vi "test-rotation2d.vi"(8 "error in (no error)":errorcluster) -> (0 "error out":errorcluster, 3 "ALL TESTS PASSED":bool)   [LabVIEW 2019]
uses:
  <vilib>/Rock Robotics/WPI/ThirdParty/JAS_Junk/TrajLib/Rotation2d_Plus.vi
  <vilib>/Rock Robotics/WPI/ThirdParty/JAS_Junk/TrajLib/MathUtil_Clamp.vi
  <vilib>/Rock Robotics/WPI/ThirdParty/JAS_Junk/TrajLib/Rotation2d_Times.vi
  <vilib>/Rock Robotics/WPI/ThirdParty/JAS_Junk/TrajLib/Util_CalcDist.vi
  <vilib>/Rock Robotics/WPI/ThirdParty/JAS_Junk/TrajLib/Rotation2d_UnaryMinus.vi
  <vilib>/Rock Robotics/WPI/ThirdParty/JAS_Junk/TrajLib/Rotation2d_CreateXY.vi
  <vilib>/Rock Robotics/WPI/ThirdParty/JAS_Junk/TrajLib/Trajectory_Library.lvlib
panel:
  out "T9 - True":bool
  out "T8 - True":bool
  out "T7 - True":bool
  out "T4 -- X -- 0":dbl
  out "T3 -- X -- 0":dbl
  out "T2 -- y -- 0":dbl
  out "T2 -- X -- 0":dbl
  out "T6 - False":bool
  out "T5 - True":bool
  out "T1 -- y -- 0":dbl
  out "T1 -- X -- 0":dbl
  out "T0 -- y -- 0":dbl
  out "T0 -- X -- 0":dbl
  # "Rotation2D Test"
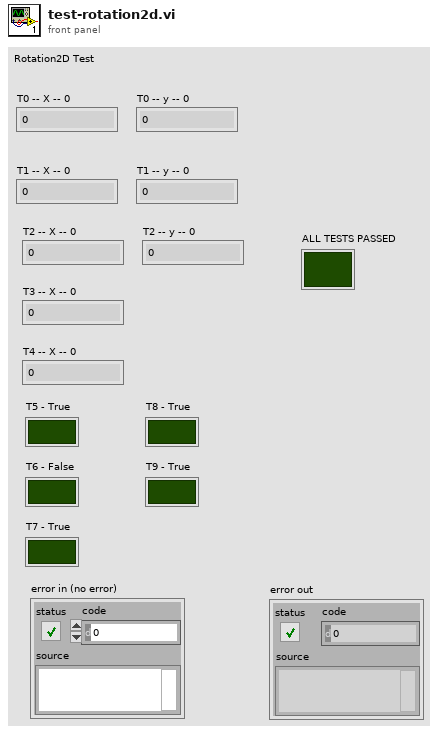
[diagram p1: front panel]
types:
  T1 = typedef "Trajectory_Library.lvlib/ROTATION2D.ctl" = cluster{"VALUE":dbl, "COS":dbl, "SIN":dbl}
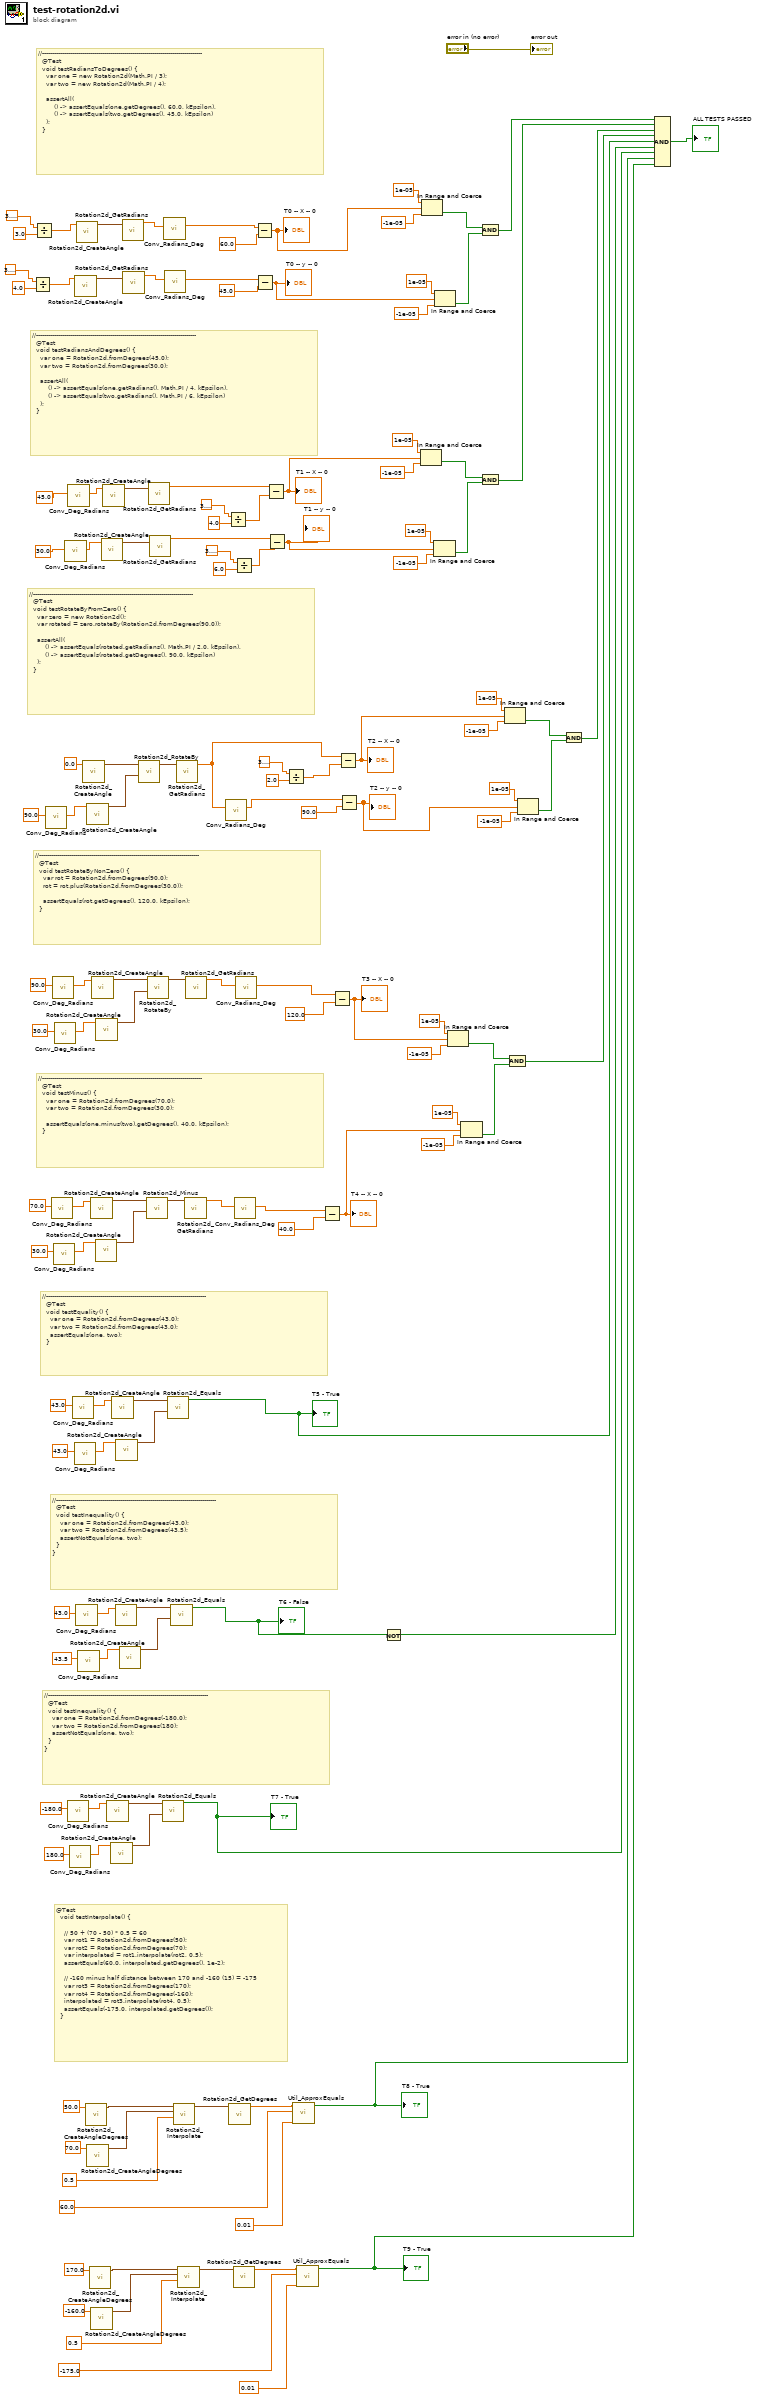
[diagram p0: block diagram]
diagram:
  # "@Test\n  void testInterpolate() {\n\n    // 50 + (70 - 50) * 0.5 = 60\n    var rot1 = Rotation2d.fromDegrees(50);\n    var rot2 = Rotation2d.fromDegrees(70);\n    var interpolated = rot1.interpolate(rot2, 0.5);\n    assertEquals(60.0, interpolated.getDegrees(), 1e-2);\n\n    // -160 minus half distance between 170 and -160 (15) = -175\n    var rot3 = Rotation2d.fromDegrees(170);\n    var rot4 = Rotation2d.fromDegrees(-160);\n    interpolated = rot3.interpolate(rot4, 0.5);\n    assertEquals(-175.0, interpolated.getDegrees());\n  }"
  # "//--------------------------------------------------------------------------------\n  @Test\n  void testInequality() {\n    var one = Rotation2d.fromDegrees(-180.0);\n    var two = Rotation2d.fromDegrees(180);\n    assertNotEquals(one, two);\n  }\n}"
  # "//--------------------------------------------------------------------------------\n  @Test\n  void testInequality() {\n    var one = Rotation2d.fromDegrees(43.0);\n    var two = Rotation2d.fromDegrees(43.5);\n    assertNotEquals(one, two);\n  }\n}"
  # "//--------------------------------------------------------------------------------\n  @Test\n  void testMinus() {\n    var one = Rotation2d.fromDegrees(70.0);\n    var two = Rotation2d.fromDegrees(30.0);\n\n    assertEquals(one.minus(two).getDegrees(), 40.0, kEpsilon);\n  }"
  # "//--------------------------------------------------------------------------------\n  @Test\n  void testRotateByNonZero() {\n    var rot = Rotation2d.fromDegrees(90.0);\n    rot = rot.plus(Rotation2d.fromDegrees(30.0));\n\n    assertEquals(rot.getDegrees(), 120.0, kEpsilon);\n  }"
  # "//--------------------------------------------------------------------------------\n  @Test\n  void testRotateByFromZero() {\n    var zero = new Rotation2d();\n    var rotated = zero.rotateBy(Rotation2d.fromDegrees(90.0));\n\n    assertAll(\n        () -> assertEquals(rotated.getRadians(), Math.PI / 2.0, kEpsilon),\n        () -> assertEquals(rotated.getDegrees(), 90.0, kEpsilon)\n    );\n  }"
  # "//--------------------------------------------------------------------------------\n  @Test\n  void testEquality() {\n    var one = Rotation2d.fromDegrees(43.0);\n    var two = Rotation2d.fromDegrees(43.0);\n    assertEquals(one, two);\n  }"
  # "//--------------------------------------------------------------------------------\n  @Test\n  void testRadiansAndDegrees() {\n    var one = Rotation2d.fromDegrees(45.0);\n    var two = Rotation2d.fromDegrees(30.0);\n\n    assertAll(\n        () -> assertEquals(one.getRadians(), Math.PI / 4, kEpsilon),\n        () -> assertEquals(two.getRadians(), Math.PI / 6, kEpsilon)\n    );\n  }"
  # "//--------------------------------------------------------------------------------\n  @Test\n  void testRadiansToDegrees() {\n    var one = new Rotation2d(Math.PI / 3);\n    var two = new Rotation2d(Math.PI / 4);\n\n    assertAll(\n        () -> assertEquals(one.getDegrees(), 60.0, kEpsilon),\n        () -> assertEquals(two.getDegrees(), 45.0, kEpsilon)\n    );\n  }"
  n1 = Divide(x=3.141592653589793, y=4.0) -> (x/y=w128:dbl)
  n2 = Divide(x=3.141592653589793, y=3.0) -> (x/y=w131:dbl)
  n3 = call <vilib>:"Conv_Deg_Radians.vi"("Degress"=90.0) -> ("Radians"=w137:dbl)  [unwired: 10 in]
  n4 = call <vilib>:"Conv_Deg_Radians.vi"("Degress"=70.0) -> ("Radians"=w82:dbl)  [unwired: 10 in]
  n5 = call <vilib>:"Conv_Deg_Radians.vi"("Degress"=90.0) -> ("Radians"=w91:dbl)  [unwired: 10 in]
  n6 = call <vilib>:"Conv_Deg_Radians.vi"("Degress"=30.0) -> ("Radians"=w89:dbl)  [unwired: 10 in]
  n7 = call <vilib>:"Conv_Deg_Radians.vi"("Degress"=30.0) -> ("Radians"=w98:dbl)  [unwired: 10 in]
  n8 = call <vilib>:"Conv_Deg_Radians.vi"("Degress"=30.0 ("y")) -> ("Radians"=w113:dbl)  [unwired: 10 in]
  n9 = call <vilib>:"Conv_Deg_Radians.vi"("Degress"=-180.0) -> ("Radians"=w63:dbl)  [unwired: 10 in]
  n10 = call <vilib>:"Conv_Deg_Radians.vi"("Degress"=45.0 ("y")) -> ("Radians"=w112:dbl)  [unwired: 10 in]
  n11 = call <vilib>:"Conv_Deg_Radians.vi"("Degress"=180.0) -> ("Radians"=w68:dbl)  [unwired: 10 in]
  n12 = call <vilib>:"Conv_Deg_Radians.vi"("Degress"=43.0) -> ("Radians"=w75:dbl)  [unwired: 10 in]
  n13 = call <vilib>:"Conv_Deg_Radians.vi"("Degress"=43.0) -> ("Radians"=w80:dbl)  [unwired: 10 in]
  n14 = call <vilib>:"Rotation2d_CreateAngle.vi"("Angle"=w128) -> ("ROTATION"=w124:T1)  [unwired: 10 in]
  n15 = call <vilib>:"Conv_Deg_Radians.vi"("Degress"=43.0) -> ("Radians"=w69:dbl)  [unwired: 10 in]
  n16 = call <vilib>:"Rotation2d_CreateAngle.vi"("Angle"=w131) -> ("ROTATION"=w127:T1)  [unwired: 10 in]
  n17 = call <vilib>:"Conv_Deg_Radians.vi"("Degress"=43.5) -> ("Radians"=w74:dbl)  [unwired: 10 in]
  n18 = call <vilib>:"Rotation2d_CreateAngle.vi"("Angle"=0.0) -> ("ROTATION"=w106:T1)  [unwired: 10 in]
  n19 = call <vilib>:"Rotation2d_CreateAngleDegrees.vi"("Angle_Degrees"=50.0) -> ("ROTATION"=w18:T1)  [unwired: 10 in]
  n20 = call <vilib>:"Rotation2d_CreateAngle.vi"("Angle"=w137) -> ("ROTATION"=w105:T1)  [unwired: 10 in]
  n21 = call <vilib>:"Rotation2d_CreateAngleDegrees.vi"("Angle_Degrees"=70.0) -> ("ROTATION"=w17:T1)  [unwired: 10 in]
  n22 = call <vilib>:"Rotation2d_CreateAngleDegrees.vi"("Angle_Degrees"=170.0) -> ("ROTATION"=w9:T1)  [unwired: 10 in]
  n23 = call <vilib>:"Rotation2d_CreateAngle.vi"("Angle"=w82) -> ("ROTATION"=w87:T1)  [unwired: 10 in]
  n24 = call <vilib>:"Rotation2d_CreateAngleDegrees.vi"("Angle_Degrees"=-160.0) -> ("ROTATION"=w8:T1)  [unwired: 10 in]
  n25 = call <vilib>:"Rotation2d_CreateAngle.vi"("Angle"=w91) -> ("ROTATION"=w96:T1)  [unwired: 10 in]
  n26 = call <vilib>:"Rotation2d_CreateAngle.vi"("Angle"=w89) -> ("ROTATION"=w86:T1)  [unwired: 10 in]
  n27 = call <vilib>:"Rotation2d_CreateAngle.vi"("Angle"=w98) -> ("ROTATION"=w95:T1)  [unwired: 10 in]
  n28 = call <vilib>:"Rotation2d_CreateAngle.vi"("Angle"=w113) -> ("ROTATION"=w120:T1)  [unwired: 10 in]
  n29 = call <vilib>:"Rotation2d_CreateAngle.vi"("Angle"=w112) -> ("ROTATION"=w121:T1)  [unwired: 10 in]
  n30 = call <vilib>:"Rotation2d_CreateAngle.vi"("Angle"=w63) -> ("ROTATION"=w66:T1)  [unwired: 10 in]
  n31 = call <vilib>:"Rotation2d_CreateAngle.vi"("Angle"=w68) -> ("ROTATION"=w65:T1)  [unwired: 10 in]
  n32 = call <vilib>:"Rotation2d_CreateAngle.vi"("Angle"=w75) -> ("ROTATION"=w78:T1)  [unwired: 10 in]
  n33 = call <vilib>:"Rotation2d_CreateAngle.vi"("Angle"=w69) -> ("ROTATION"=w72:T1)  [unwired: 10 in]
  n34 = call <vilib>:"Rotation2d_CreateAngle.vi"("Angle"=w80) -> ("ROTATION"=w77:T1)  [unwired: 10 in]
  n35 = call <vilib>:"Rotation2d_CreateAngle.vi"("Angle"=w74) -> ("ROTATION"=w71:T1)  [unwired: 10 in]
  n36 = call <vilib>:"Rotation2d_GetRadians.vi"("in ROTATION"=w127) -> ("AngleRadians"=w126:dbl)  [unwired: 10 in]
  n37 = call <vilib>:"Rotation2d_GetRadians.vi"("in ROTATION"=w124) -> ("AngleRadians"=w125:dbl)  [unwired: 10 in]
  n38 = call <vilib>:"Rotation2d_RotateBy.vi"("other Rotation"=w105, "in ROTATION"=w106) -> ("out ROTATION"=w104:T1)  [unwired: 9 in]
  n39 = call <vilib>:"Rotation2d_Minus.vi"("other ROTATION"=w86, "in ROTATION"=w87) -> ("out ROTATION"=w85:T1)  [unwired: 9 in]
  n40 = call <vilib>:"Rotation2d_RotateBy.vi"("other Rotation"=w95, "in ROTATION"=w96) -> ("out ROTATION"=w94:T1)  [unwired: 9 in]
  n41 = call <vilib>:"Rotation2d_GetRadians.vi"("in ROTATION"=w121) -> ("AngleRadians"=w109:dbl)  [unwired: 10 in]
  n42 = call <vilib>:"Rotation2d_GetRadians.vi"("in ROTATION"=w120) -> ("AngleRadians"=w108:dbl)  [unwired: 10 in]
  n43 = call <vilib>:"Rotation2d_Equals.vi"("other ROTATION"=w65, "in ROTATION"=w66) -> ("Equals"=w22:bool)  [unwired: 9 in]
  "T7 - True" <- w22
  n44 = call <vilib>:"Conv_Radians_Deg.vi"("Radians"=w126) -> ("Degrees"=w123:dbl)  [unwired: 10 in]
  n45 = call <vilib>:"Conv_Radians_Deg.vi"("Radians"=w125) -> ("Degrees"=w122:dbl)  [unwired: 10 in]
  n46 = call <vilib>:"Rotation2d_Equals.vi"("other ROTATION"=w77, "in ROTATION"=w78) -> ("Equals"=w24:bool)  [unwired: 9 in]
  "T5 - True" <- w24
  n47 = call <vilib>:"Rotation2d_Equals.vi"("other ROTATION"=w71, "in ROTATION"=w72) -> ("Equals"=w25:bool)  [unwired: 9 in]
  "T6 - False" <- w25
  n48 = call <vilib>:"Rotation2d_Interpolate.vi"("T"=0.5, "EncValue ROTATION"=w17, "in ROTATION"=w18) -> ("Interpolated ROTATION"=w15:T1)  [unwired: 8 in]
  n49 = call <vilib>:"Rotation2d_GetRadians.vi"("in ROTATION"=w104) -> ("AngleRadians"=w100:dbl)  [unwired: 10 in]
  n50 = call <vilib>:"Rotation2d_Interpolate.vi"("T"=0.5, "EncValue ROTATION"=w8, "in ROTATION"=w9) -> ("Interpolated ROTATION"=w6:T1)  [unwired: 8 in]
  n51 = call <vilib>:"Rotation2d_GetRadians.vi"("in ROTATION"=w85) -> ("AngleRadians"=w84:dbl)  [unwired: 10 in]
  n52 = call <vilib>:"Rotation2d_GetRadians.vi"("in ROTATION"=w94) -> ("AngleRadians"=w93:dbl)  [unwired: 10 in]
  n53 = call <vilib>:"Conv_Radians_Deg.vi"("Radians"=w100) -> ("Degrees"=w99:dbl)  [unwired: 10 in]
  n54 = Divide(x=3.141592653589793, y=4.0) -> (x/y=w114:dbl)
  n55 = call <vilib>:"Rotation2d_GetDegrees.vi"("in ROTATION"=w15) -> ("AngleDegrees"=w14:dbl)  [unwired: 10 in]
  n56 = Divide(x=3.141592653589793, y=6.0) -> (x/y=w115:dbl)
  n57 = call <vilib>:"Rotation2d_GetDegrees.vi"("in ROTATION"=w6) -> ("AngleDegrees"=w5:dbl)  [unwired: 10 in]
  n58 = call <vilib>:"Conv_Radians_Deg.vi"("Radians"=w84) -> ("Degrees"=w81:dbl)  [unwired: 10 in]
  n59 = call <vilib>:"Conv_Radians_Deg.vi"("Radians"=w93) -> ("Degrees"=w90:dbl)  [unwired: 10 in]
  n60 = Subtract(x=w123, y=60.0) -> (x-y=w56:dbl)
  "T0 -- X -- 0" <- w56
  n61 = Subtract(x=w122, y=45.0) -> (x-y=w55:dbl)
  "T0 -- y -- 0" <- w55
  n62 = Subtract(x=w109, y=w114) -> (x-y=w45:dbl)
  "T1 -- X -- 0" <- w45
  n63 = Subtract(x=w108, y=w115) -> (x-y=w46:dbl)
  "T1 -- y -- 0" <- w46
  n64 = Divide(x=3.141592653589793, y=2.0) -> (x/y=w101:dbl)
  n65 = call <vilib>:"Util_ApproxEquals.vi"("Tolerance"=0.01, "Value 2"=60.0, "Value 1"=w14) -> ("ApproxEquals"=w2:bool)  [unwired: 8 in]
  "T8 - True" <- w2
  n66 = call <vilib>:"Util_ApproxEquals.vi"("Tolerance"=0.01, "Value 2"=-175.0, "Value 1"=w5) -> ("ApproxEquals"=w1:bool)  [unwired: 8 in]
  "T9 - True" <- w1
  n67 = Subtract(x=w81, y=40.0 ("x")) -> (x-y=w27:dbl)
  "T4 -- X -- 0" <- w27
  n68 = Subtract(x=w90, y=120.0 ("x")) -> (x-y=w28:dbl)
  "T3 -- X -- 0" <- w28
  n69 = Subtract(x=w100, y=w101) -> (x-y=w37:dbl)
  "T2 -- X -- 0" <- w37
  n70 = Subtract(x=w99, y=90.0) -> (x-y=w36:dbl)
  "T2 -- y -- 0" <- w36
  n71 = Not(x=w25) -> (.not. x?=w23:bool)
  n72 = In Range and Coerce(upper limit=1e-05, x=w45, lower limit=-1e-05) -> (In Range?=w48:bool)  [unwired: 1 out]
  n73 = In Range and Coerce(upper limit=1e-05, x=w56, lower limit=-1e-05) -> (In Range?=w58:bool)  [unwired: 1 out]
  n74 = In Range and Coerce(upper limit=1e-05, x=w46, lower limit=-1e-05) -> (In Range?=w47:bool)  [unwired: 1 out]
  n75 = In Range and Coerce(upper limit=1e-05, x=w55, lower limit=-1e-05) -> (In Range?=w57:bool)  [unwired: 1 out]
  n76 = In Range and Coerce(upper limit=1e-05, x=w28, lower limit=-1e-05) -> (In Range?=w30:bool)  [unwired: 1 out]
  n77 = In Range and Coerce(upper limit=1e-05, x=w27, lower limit=-1e-05) -> (In Range?=w29:bool)  [unwired: 1 out]
  n78 = And(x=w48, y=w47) -> (x .and. y?=w44:bool)
  n79 = And(x=w58, y=w57) -> (x .and. y?=w53:bool)
  n80 = In Range and Coerce(upper limit=1e-05, x=w37, lower limit=-1e-05) -> (In Range?=w39:bool)  [unwired: 1 out]
  n81 = And(x=w30, y=w29) -> (x .and. y?=w26:bool)
  n82 = In Range and Coerce(upper limit=1e-05, x=w36, lower limit=-1e-05) -> (In Range?=w38:bool)  [unwired: 1 out]
  n83 = And(x=w39, y=w38) -> (x .and. y?=w35:bool)
  n84 = Compound Arithmetic op=AND(w53, w44, w35, w26, w24, w23, w22, w2, w1) -> (→"ALL TESTS PASSED":bool)
  "error out" <- "error in (no error)"
